vi "ProdaNG.Tree.Results.Update.vi"(5 "Identification":T2, 6 "Products":T1[](array[typedef]), 7 "TreeControl in":refnum<vi>, 8 "error in (no error)":errorcluster, 11 "dbHandle in":i32) -> (0 "error out":errorcluster, 2 "Number of Rows":i32, 3 "dbHandle out":i32)   [LabVIEW 2016]
uses:
  Controls/ProdaNG.Product.ctl
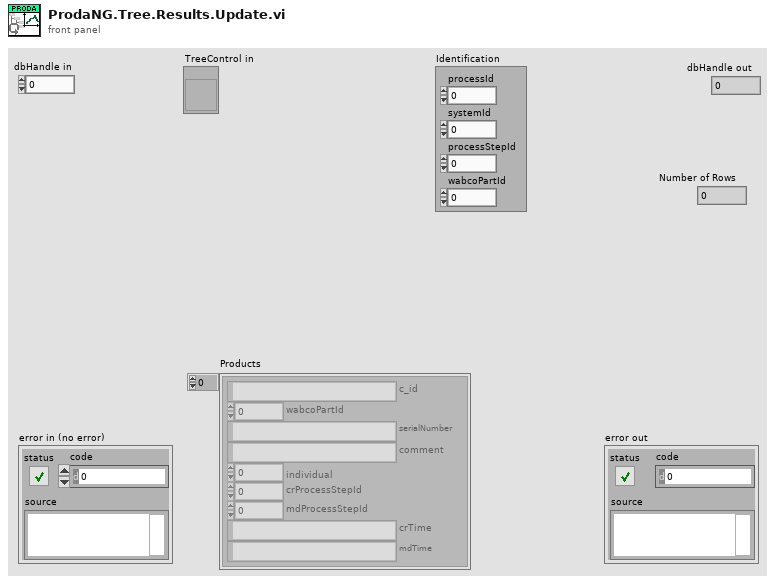
[diagram p1: front panel]
types:
  T1 = typedef "ProdaNG.Product.ctl" = cluster{"c_id":string, "wabcoPartId":i32, "serialNumber":string, "comment":string, "individual":i32, "crProcessStepId":i32, "mdProcessStepId":i32, "crTime":string, "mdTime":string}
  T2 = cluster{"processId":i32, "systemId":i32, "processStepId":i32, "wabcoPartId":i32}
  T3 = typedef "ProdaNG.UnitSimple.ctl" = cluster{"name":string, "i_id":i32}
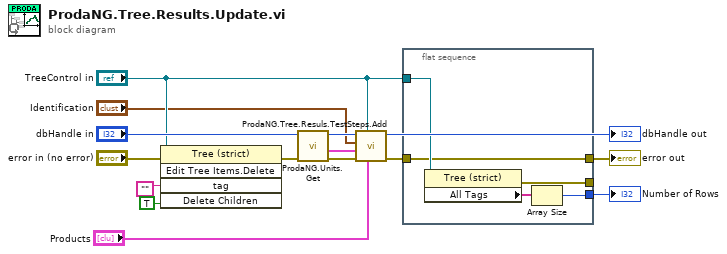
[diagram p0: block diagram]
diagram:
  n1 = invoke on="Invoke Node" class="Tree (strict)" method="Edit Tree Items.Delete"(reference="TreeControl in", error in="error in (no error)", "tag"="", "Delete Children"=TRUE ("Delete Children?")) -> (error out=w5:errorcluster)  [unwired: 1 in, 4 out]
  n2 = call "ProdaNG.Units.Get.vi"("error in (no error)"=w5, "dbHandleIn"="dbHandle in") -> ("error out"=w4:errorcluster, "units simple"=w10:T3[], "dbHandle"=w9:i32)  [unwired: 6 in, 1 out]
  n3 = call "ProdaNG.Tree.Resuls.TestSteps.Add.vi"("Products"="Products", "TestStepsTree"="TreeControl in", "error in (no error)"=w4, "units"=w10, "Identification"="Identification", "dbHandleIn"=w9) -> ("error out"=w13:errorcluster, "dbHandle"=→"dbHandle out":i32)  [unwired: 4 in]
  n4 = flat-sequence {
    tunnel: w13 -> [w18]
    tunnel: "TreeControl in" -> [w20]
    tunnel: [w18] -> w12
    tunnel: [w16] -> w11
    tunnel: [w17] -> _
    frame #0 {
      n5 = property class="Tree (strict)"(reference=w20) -> (error out=w17:errorcluster, "All Tags"=w19:string[])  [unwired: 1 in, 1 out]
      n6 = Array Size(array=w19) -> (size(s)=w16:i32)
    }
  }
  "error out" <- w12
  "Number of Rows" <- w11
